vi "Set All Enpoint Configurations.vi"(8 "error in (no error)":errorcluster, 10 "All Endpoint Configurations":T1[](array[typedef]), 11 "Endpoint Config Section Ref in":T3 format="%.0x") -> (0 "error out":errorcluster, 3 "Endpoint Config Section Ref out":T3 format="%.0x")   [LabVIEW 2017, in "SLSC Switch Scripting.lvlib"]
uses:
  SLSC Switch Scripting.lvlib
  <vilib>/NI Veristand/Custom Device API/Custom Device Item Ref.ctl
  Endpoint Configuration Cluster.ctl
  Endpoint Configuration Enum.ctl
  <vilib>/NI VeriStand/Custom Device API/Custom Device API.lvlib
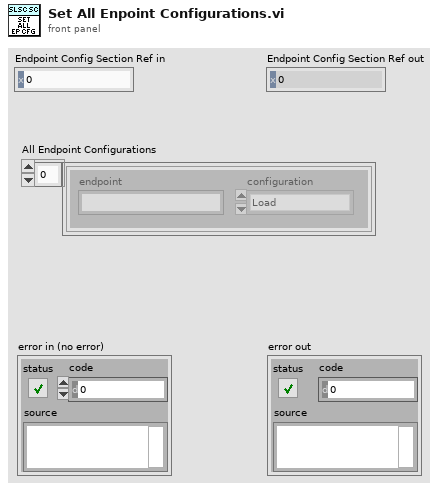
[diagram p1: front panel]
types:
  T1 = typedef "SLSC Switch Scripting.lvlib/Endpoint Configuration Cluster.ctl" = cluster{"endpoint":string, "configuration":T2}
  T2 = typedef "SLSC Switch Scripting.lvlib/Endpoint Configuration Enum.ctl" = enum16{"Load", "Source", "Configuration"}
  T3 = typedef "Custom Device API.lvlib/Custom Device Item Ref.ctl" = u64
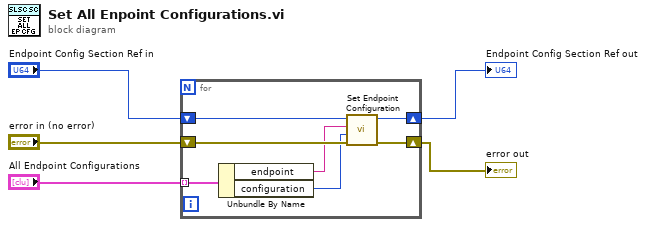
[diagram p0: block diagram]
diagram:
  n1 = for {
    shift-right: [w9] -> w4
    shift-left: "error in (no error)" -> [w10]
    shift-right: [w11] -> w2
    shift-left: "Endpoint Config Section Ref in" -> [w12]
    tunnel: "All Endpoint Configurations" -> [w8] mode=indexing
    n2 = Unbundle By Name(w8) -> ("endpoint"=w7:string, "configuration"=w6:T2)
    n3 = call "Set Endpoint Configuration.vi"("error in (no error)"=w10, "Configuration Type"=w6, "Endpoint"=w7, "Endpoint Config Section Ref in"=w12) -> ("error out"=w9:errorcluster, "Endpoint Config Section Ref in"=w11:T3)  [unwired: 6 in]
  }
  "error out" <- w4
  "Endpoint Config Section Ref out" <- w2
